vi "Target3.vi"() -> ()   [LabVIEW 2025]
uses:
  <vilib>/Platform/TimedLoop/XDataNode/wakeup.ctl
  <vilib>/Platform/TimedLoop/XDataNode/XDNodeRunTimeDep.lvlib
  <vilib>/Platform/TimedLoop/XDataNode/nitl_modes.ctl
  <vilib>/Platform/TimedLoop/XDataNode/timing_clust.ctl
  <vilib>/platform/TimedLoop/XDataNode/XDataNode.xnode
  <vilib>/rvi/linearAlgebra/MatrixMultiply/XNode/nifxpla_MatrixMultiply.xnode
  <vilib>/rvi/linearAlgebra/MatrixMultiply/simVIs/nifxpla_MatrixMultiply_SimTemplateEinEout.vi
  <vilib>/rvi/linearAlgebra/MatrixMultiply/simVIs/nifxpla_MatrixMultiply_SimTemplateEinVout.vi
  <vilib>/rvi/linearAlgebra/MatrixMultiply/simVIs/nifxpla_MatrixMultiply_SimTemplateVinEout.vi
  <vilib>/rvi/linearAlgebra/MatrixMultiply/simVIs/nifxpla_MatrixMultiply_SimTemplateVinVout.vi
  <vilib>/rvi/DataTransferAndStorage/Container/XNode/niFpgaContainer.xnode
  <vilib>/rvi/interface/RandomDataEmulation/nirviRandomDataFpgaMultiElementTemplate.vi
  <vilib>/rvi/interface/RandomDataEmulation/nirviRandomDataFpgaReadWriteTemplate.vi
panel:
  out "operation overflow":bool
  out "Array 4":fxp<+/-,32,16>[](array[numeric])
  out "Array 5":fxp<+/-,32,16>[](array[numeric])
  out "Array 2":bool[](array[boolean])
  out "Array":bool[](array[boolean])
  out "output valid":bool
  out "Ready for Input":bool
  out "Numeric":i32
  out "Numeric 2":i32
  out "appended array":fxp<+/-,32,16>[](array[numeric])
  out "appended array 2":fxp<+/-,32,16>[](array[numeric])
  out "Array 3":fxp<+/-,32,16>[](array[numeric])
  out "cr":fxp<+/-,32,16>[](array[numeric])
  out "element":fxp<+/-,32,16>
  out "element 2":fxp<+/-,32,16>
  out "ready for a":bool[](array[boolean])
  out "And 1":bool[](array[boolean])
  out "ready for b":bool[](array[boolean])
  out "And 2":bool[](array[boolean])
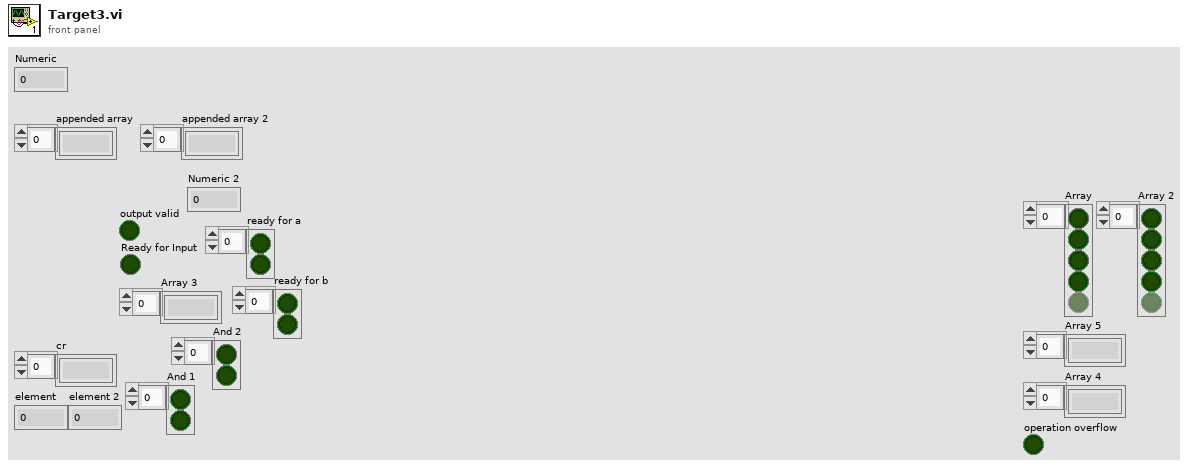
[diagram p1: front panel]
types:
  T1 = typedef "XDNodeRunTimeDep.lvlib/timing_clust.ctl" = cluster{"Expected End [f-1]":u64, "Actual End [f-1]":u64, "Finished Late? [f-1]":bool, "Expected End [i-1]":u64, "Actual End [i-1]":u64, "Finished Late? [i-1]":bool, "Expected Start [i]":u64, "Actual Start [i]":u64, "Expected Start [f]":u64, "Actual Start [f]":u64, "Source Name":string, "Structure Name":string, "Period":i64, "Deadline":i64, "Offset":i64, "Start":i64, "Priority":i32, "Timeout":i32, "Mode":T2, "Wakeup Reason":T3, "Error":errorcluster, "Source Type":string, "Secondary Source Type":string, "Global End Time":u64, "Global Start Time":u64, "Frame Duration":u64, "Iteration Duration":u64, "Assigned CPU":i32, "I/O Scan Engine Mode":u32}
  T2 = typedef "XDNodeRunTimeDep.lvlib/nitl_modes.ctl" = enum32{"No Change", "Process missed periods, maintain original phase", "Discard missed periods, maintain original phase", "Process missed periods, ignore original phase", "Discard missed periods, ignore original phase"}
  T3 = typedef "XDNodeRunTimeDep.lvlib/wakeup.ctl" = enum32{"Normal", "Aborted", "Asynchronous wakeup", "Timing source error", "Timed loop error", "Timeout"}
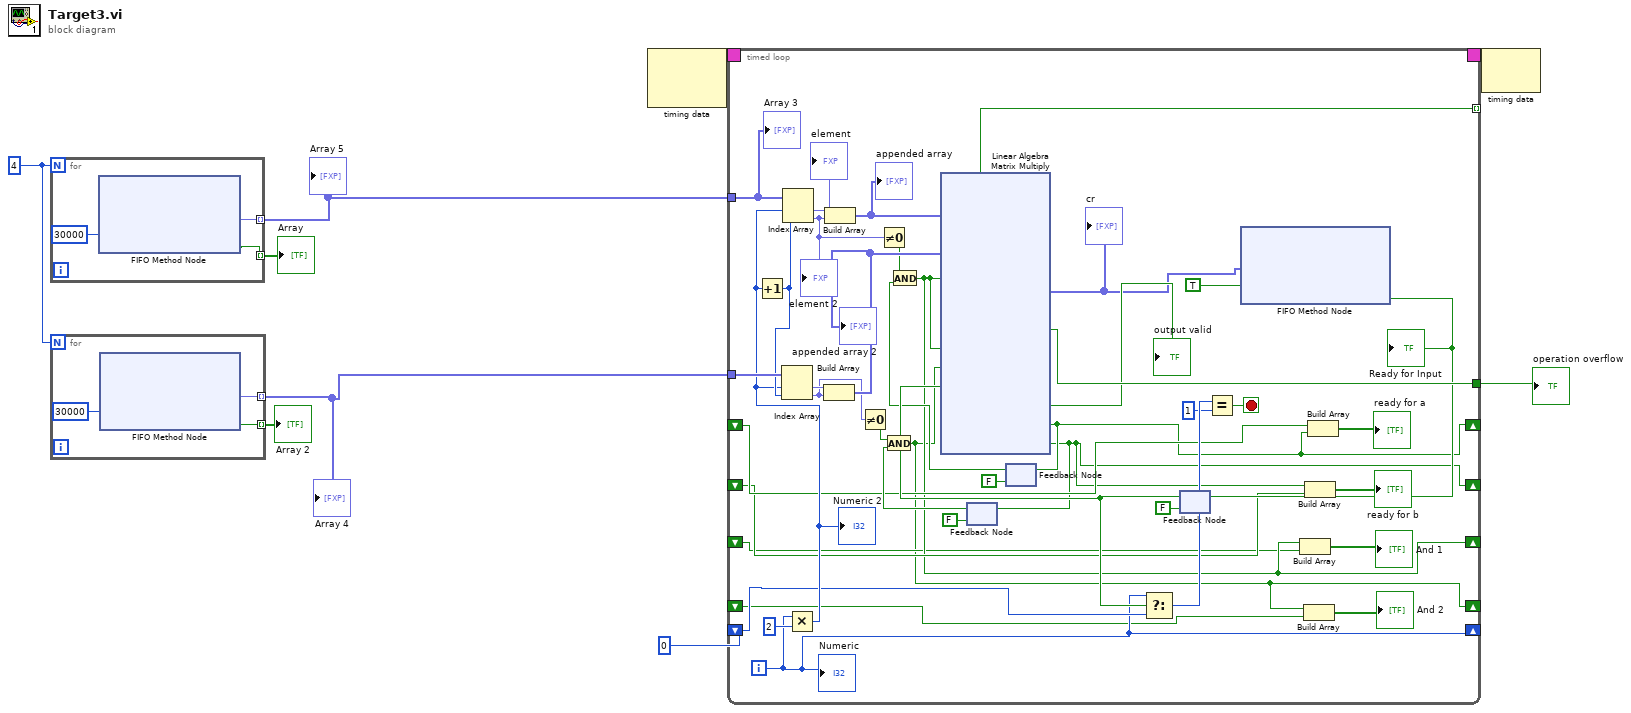
[diagram p0: block diagram]
diagram:
  w7 = 4
  n1 = for {
    N: w7 -> [_]
    tunnel: [w12] -> w3 mode=indexing
    tunnel: [w10] -> w6 mode=indexing
    n2 = xnode ("FIFO Method Node")("Timeout"=30000) -> ("Element"=w12:fxp<+/-,32,16>, "Timed Out?"=w10:bool)  [unwired: 1 in, 1 out]
  }
  "Array" <- w6
  "Array 5" <- w3
  n3 = for {
    N: w7 -> [_]
    tunnel: [w15] -> w2 mode=indexing
    tunnel: [w13] -> w5 mode=indexing
    n4 = xnode ("FIFO Method Node")("Timeout"=30000) -> ("Element"=w15:fxp<+/-,32,16>, "Timed Out?"=w13:bool)  [unwired: 1 in, 1 out]
  }
  "Array 2" <- w5
  "Array 4" <- w2
  n5 = node-c288() -> (w9:T1)  [unwired: 2 in]
  n6 = timed-loop {
    timing: w9 -> [_]
    timing-out: [_] -> w8
    tunnel: w3 -> [w39]
    tunnel: w2 -> [w54]
    tunnel: [w46] -> w4
    shift-right: [w35] -> _
    shift-left: 0 -> [w36]
    tunnel: [w19] -> _ mode=indexing
    shift-right: [w26] -> _
    shift-left: _ -> [w27]
    shift-right: [w21] -> _
    shift-left: _ -> [w20]
    shift-right: [w19] -> _
    shift-left: _ -> [w18]
    shift-right: [w16] -> _
    shift-left: _ -> [w17]
    i -> [w35]
    stop <- w50 stop-if-true
    n7 = Multiply(x=w35, y=2) -> (x*y=w37:i32)
    "Numeric 2" <- w37
    n8 = Increment(x=w37) -> (x+1=w43:i32)
    n9 = Index Array(array=w54, index #1=w37, index #2=w43) -> (element #1=w55:fxp<+/-,32,16>, element #2=w33:fxp<+/-,32,16>)
    n10 = Index Array(array=w39, index #1=w37, index #2=w43) -> (element #1=w56:fxp<+/-,32,16>, element #2=w28:fxp<+/-,32,16>)
    "element" <- w56
    "element 2" <- w28
    n11 = Build Array(w55, w33) -> (w34:fxp<+/-,32,16>[])
    "appended array 2" <- w34
    n12 = Build Array(w56, w28) -> (w40:fxp<+/-,32,16>[])
    "appended array" <- w40
    n13 = Not Equal To 0?(x=w33) -> (x != 0?=w32:bool)
    n14 = Not Equal To 0?(x=w28) -> (x != 0?=w30:bool)
    n15 = feedback #1(FALSE ("ready for b")) -> (w31:bool)
    n16 = And(x=w32, y=w31) -> (x .and. y?=w16:bool)
    n17 = feedback #2(FALSE ("ready for a")) -> (w29:bool)
    n18 = And(x=w30, y=w29) -> (x .and. y?=w19:bool)
    n19 = feedback #3(FALSE ("Ready for Input")) -> (w51:bool)
    n20 = xnode ("Linear Algebra Matrix Multiply")("ar"=w40, "br"=w34, "a valid"=w19, "b valid"=w16, "ready for output (T)"=w51) -> ("cr"=w41:fxp<+/-,32,16>[], "operation overflow"=w46:bool, "output valid"=→"output valid":bool, "ready for a"=w26:bool, "ready for b"=w21:bool)  [unwired: 2 in, 1 out]
    "cr" <- w41
    n21 = feedback-in #1(w21) -> ()
    n22 = feedback-in #2(w26) -> ()
    n23 = Select(t=w35, s=w51, f=w36) -> (s? t:f=w49:i32)
    n24 = Equal?(x=w49, y=1) -> (x = y?=w50:bool)
    n25 = xnode ("FIFO Method Node")("Element"=w41, "Input Valid"=TRUE) -> ("Ready for Input"=w45:bool)  [unwired: 1 in, 1 out]
    "Ready for Input" <- w45
    n26 = feedback-in #3(w45) -> ()
    n27 = Build Array(w19, w18) -> (→"And 1":bool[])
    n28 = Build Array(w16, w17) -> (→"And 2":bool[])
    n29 = Build Array(w21, w20) -> (→"ready for b":bool[])
    n30 = Build Array(w27, w26) -> (→"ready for a":bool[])
    "Numeric" <- w35
    "Array 3" <- w39
  }
  "operation overflow" <- w4
  n31 = node-c288(w8) -> ()  [unwired: 1 out]
